vi "Hysteresis Cross Point Detection.vi"(6 "sampling frequency [Hz]":dbl=11025.0, 8 "init state":bool=TRUE, 9 "lower threshold (0)":dbl format="%.2f", 10 "upper threshold (0)":dbl format="%.2f", 11 "x[n]":dbl[](array[numeric]) format="%.2f") -> (0 "final state":bool, 2 "falling edges [s]":dbl[](array[numeric]) format="%.2f", 3 "rising edges [s]":dbl[](array[numeric]) format="%.2f")   [LabVIEW 2017, in "SoundVib_TachProcess.lvlib"]
doc: "Detects the rising and falling edges of the tachometer pulses contained in <B>x[n]</B>."
uses:
  <vilib>/addons/Sound and Vibration/Order Analysis/Tach Process/SoundVib_TachProcess.lvlib
panel:
  # "Cross Point Detection"
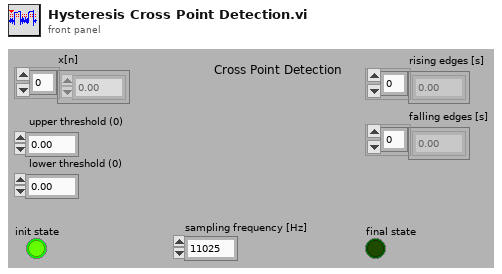
[diagram p1: front panel]
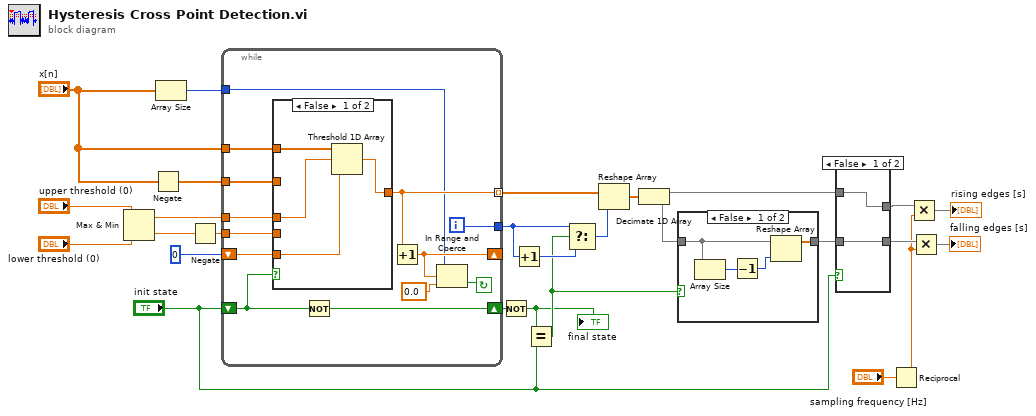
[diagram p0: block diagram]
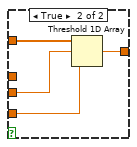
[diagram p2: hidden frame]
diagram:
  n1 = Max & Min(x="upper threshold (0)", y="lower threshold (0)") -> (max(x,y)=w7:dbl, min(x,y)=w12:dbl)
  n2 = Negate(x="x[n]") -> (-x=w24:dbl[])
  n3 = Array Size(array="x[n]") -> (size(s)=w13:i32)
  n4 = Negate(x=w12) -> (-x=w11:dbl)
  n5 = while {
    tunnel: w13 -> [w30]
    tunnel: [w32] -> w21
    tunnel: w7 -> [w34]
    tunnel: [w33] -> w23 mode=indexing
    tunnel: w11 -> [w37]
    tunnel: w24 -> [w38]
    tunnel: "x[n]" -> [w35]
    shift-left: 0 -> [w36]
    shift-right: [w31] -> _
    shift-left: "init state" -> [w39]
    shift-right: [w40] -> w10
    i -> [w32]
    stop <- w29 continue-if-true
    n6 = case shown="False" w39 {
      tunnel: w38 -> [_ w48]
      tunnel: w37 -> [_ w47]
      tunnel: w36 -> [w42 w46]
      tunnel: [w41 w45] -> w33
      tunnel: w35 -> [w44 _]
      tunnel: w34 -> [w43 _]
      frame False {
        n7 = Threshold 1D Array(1:w42, 2:w43, 3:w44) -> (0:w41:dbl)
      }
      frame True {
        n8 = Threshold 1D Array(1:w46, 2:w47, 3:w48) -> (0:w45:dbl)
      }
    }
    n9 = Not(x=w39) -> (.not. x?=w40:bool)
    n10 = Increment(x=w33) -> (x+1=w31:dbl)
    n11 = In Range and Coerce(upper limit=w30, x=w31, lower limit=0.0) -> (In Range?=w29:bool)  [unwired: 1 out]
  }
  n12 = Not(x=w10) -> (.not. x?=w9:bool)
  "final state" <- w9
  n13 = Increment(x=w21) -> (x+1=w22:i32)
  n14 = Equal?(x=w9, y="init state") -> (x = y?=w18:bool)
  n15 = Select(t=w21, s=w18, f=w22) -> (s? t:f=w20:i32)
  n16 = Reshape Array(w23, w20) -> (w19:dbl[])
  n17 = Decimate 1D Array(w19) -> (w15:dbl[], w14:dbl[])
  n18 = case shown="False" w18 {
    tunnel: w14 -> [w50 w53]
    tunnel: [w49 w53] -> w17
    frame False {
      n19 = Array Size(array=w50) -> (size(s)=w52:i32)
      n20 = Decrement(x=w52) -> (x-1=w51:i32)
      n21 = Reshape Array(w50, w51) -> (w49:dbl[])
    }
    frame True {
    }
  }
  n22 = case shown="False" "init state" {
    tunnel: w17 -> [w54 w56]
    tunnel: w15 -> [w55 w57]
    tunnel: [w54 w57] -> w4
    tunnel: [w55 w56] -> w5
    frame False {
    }
    frame True {
    }
  }
  n23 = Reciprocal(x="sampling frequency [Hz]") -> (1/x=w3:dbl)
  n24 = Multiply(x=w5, y=w3) -> (x*y=→"rising edges [s]":dbl[])
  n25 = Multiply(x=w4, y=w3) -> (x*y=→"falling edges [s]":dbl[])
